vi "USB send low.vi"(4 "Error in":errorcluster, 5 "bytes to read":u32=8, 6 "Tx msg cluster":T1={"addr"=1, "cmd"="A", "data (float)"=0.0}, 7 "Port":refnum<visa-resource-name>) -> (0 "Error out":errorcluster, 2 "Data returned":string, 3 "Port out":refnum<visa-resource-name>)   [LabVIEW 2017]
uses:
  ctls/USB Tx msg cluster.ctl
panel:
  out "Bytes returned":u32
  out "Write buffer":string
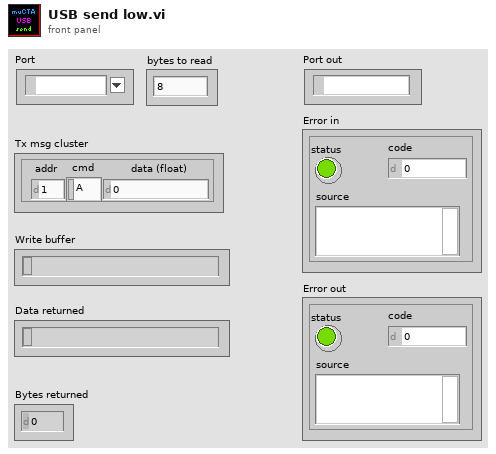
[diagram p1: front panel]
types:
  T1 = typedef "USB Tx msg cluster.ctl" = cluster{"addr":u8, "cmd":string, "data (float)":sgl}
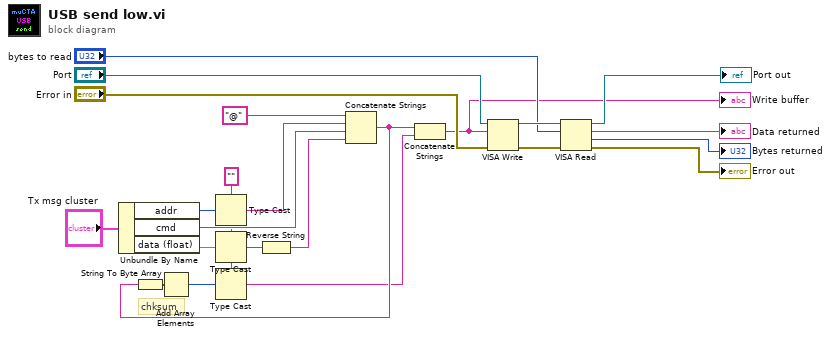
[diagram p0: block diagram]
diagram:
  w4 = ""
  # "chksum"
  n1 = Unbundle By Name("Tx msg cluster") -> ("addr"=w17:u8, "cmd"=w9:string, "data (float)"=w16:sgl)
  n2 = Type Cast(type=w4, x=w17) -> (*(type *) &x=w10:string)
  n3 = Type Cast(type=w4, x=w16) -> (*(type *) &x=w8:string)
  n4 = Reverse String(1:w8) -> (0:w1:string)
  n5 = Concatenate Strings("@", w10, w9, w1) -> (w6:string)
  n6 = String To Byte Array(string=w6) -> (unsigned byte array=w5:u8[])
  n7 = Add Array Elements(numeric array=w5) -> (sum=w3:u8)
  n8 = Type Cast(type=w4, x=w3) -> (*(type *) &x=w2:string)
  n9 = Concatenate Strings(w6, w2) -> (w7:string)
  "Write buffer" <- w7
  n10 = VISA Write(VISA resource name="Port", write buffer=w7, error in (no error)="Error in") -> (VISA resource name out=w19:refnum<visa-resource-name>, error out=w22:errorcluster)  [unwired: 1 out]
  n11 = VISA Read(VISA resource name=w19, byte count="bytes to read", error in (no error)=w22) -> (VISA resource name out=→"Port out":refnum<visa-resource-name>, read buffer=→"Data returned":string, return count=→"Bytes returned":u32, error out=→"Error out":errorcluster)
